vi "Gas Thermal Target Temperatures.vi"(8 "error in (no error)":errorcluster, 10 "Target RTDout-RTDin in":dbl, 11 "Inlet Temperature (F) - Target in":dbl) -> (0 "error out":errorcluster, 1 "Target RTDout-RTDin out":dbl, 2 "Target RTDout":dbl, 3 "Target Inlet Temperature (F)":dbl)   [LabVIEW 2019]
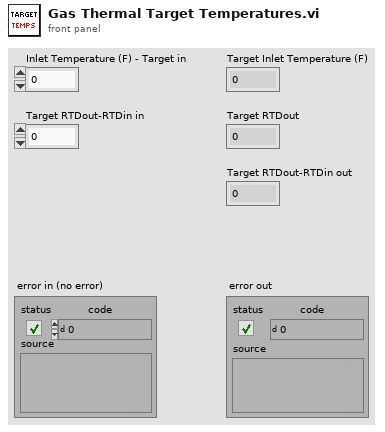
[diagram p1: front panel]
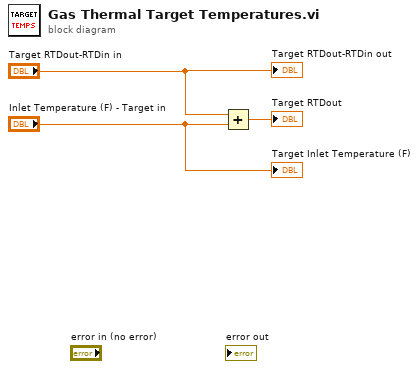
[diagram p0: block diagram]
diagram:
  n1 = Add(x="Target RTDout-RTDin in", y="Inlet Temperature (F) - Target in") -> (x+y=→"Target RTDout":dbl)
  "Target RTDout-RTDin out" <- "Target RTDout-RTDin in"
  "Target Inlet Temperature (F)" <- "Inlet Temperature (F) - Target in"
